vi "_Parse Reliability List.vi"(0 "Input String":string) -> (1 "Reliability List":i32[](array[numeric]), 2 "Reliability out":i32)   [LabVIEW 2020, in "Rohde&Schwarz CMWXP NR FR1 Measurement.lvlib"]
uses:
  <instrlib>/Rohde&Schwarz CMWXP NR FR1 Measurement/Rohde&Schwarz CMWXP NR FR1 Measurement.lvlib
  <instrlib>/Rohde&Schwarz CMWXP NR FR1 Measurement/Private/rsidr_core.llb/rsidr_core.lvlib
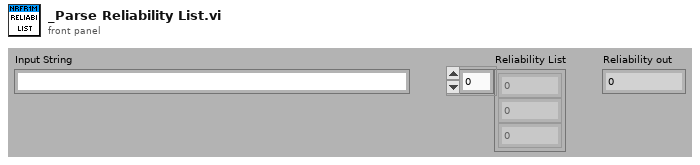
[diagram p1: front panel]
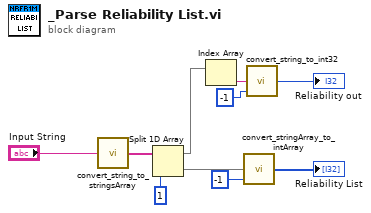
[diagram p0: block diagram]
diagram:
  n1 = call <instrlib>:"convert_string_to_stringsArray.vi"("String in"="Input String") -> ("string array out"=w1:string[])  [unwired: 3 in, 1 out]
  n2 = Split 1D Array(array=w1, index=1) -> (first subarray=w9:string[], second subarray=w5:string[])
  n3 = Index Array(array=w9) -> (element=w7:string)  [unwired: 1 in]
  n4 = call <instrlib>:"convert_stringArray_to_intArray.vi"("default (0)"=-1, "string array in"=w5) -> ("int32 array out"=→"Reliability List":i32[])  [unwired: 3 in]
  n5 = call <instrlib>:"convert_string_to_int32.vi"("default (0)"=-1 ("default (0 I32)"), "String in"=w7) -> ("int32 value out"=→"Reliability out":i32)  [unwired: 3 in]
